vi "Single Sweep.vi"() -> ()   [LabVIEW 2016]
uses:
  Keithley 2600 Series/Public/Channel.ctl
  Keithley 2600 Series/Keithley 2600 Series.lvlib
panel:
  out "error out":errorcluster
  out "Data Array Out":dbl[](array[numeric])
  in  "End (V)":dbl
  in  "Start (V)":dbl
  in  "Current Limit (A)":dbl=0.1
  in  "Step Numbers":u32=1
  in  "VISA resource name":refnum<visa-resource-name>
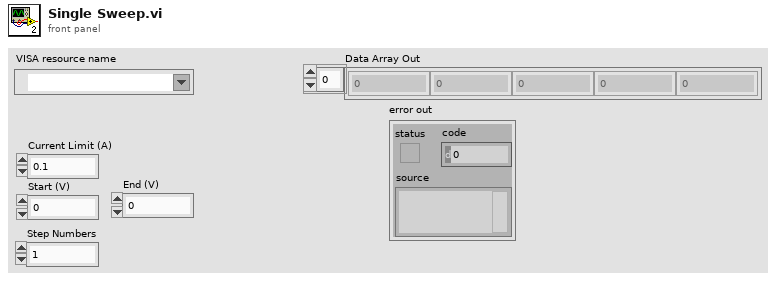
[diagram p1: front panel]
types:
  T1 = enum32{"Normal", "Big Endian", "Little Endian", "Network", "Swapped"}
  T2 = enum32{"ASCII", "Real 32", "Real 64", "Single Precision Real", "Double Precision Real"}
  T3 = enum16{"Current", "Voltage", "IV", "Resistance", "Power"}
  T4 = enum16{"Linear Current", "Linear Voltage", "Logarithimic Current", "Logarithimic Voltage", "List Current", "List Voltage"}
  T5 = typedef "Keithley 2600 Series.lvlib/Channel.ctl" = enum32{"Channel A", "Channel B"}
  T6 = enum32{"Current", "Voltage", "Resistance", "Power"}
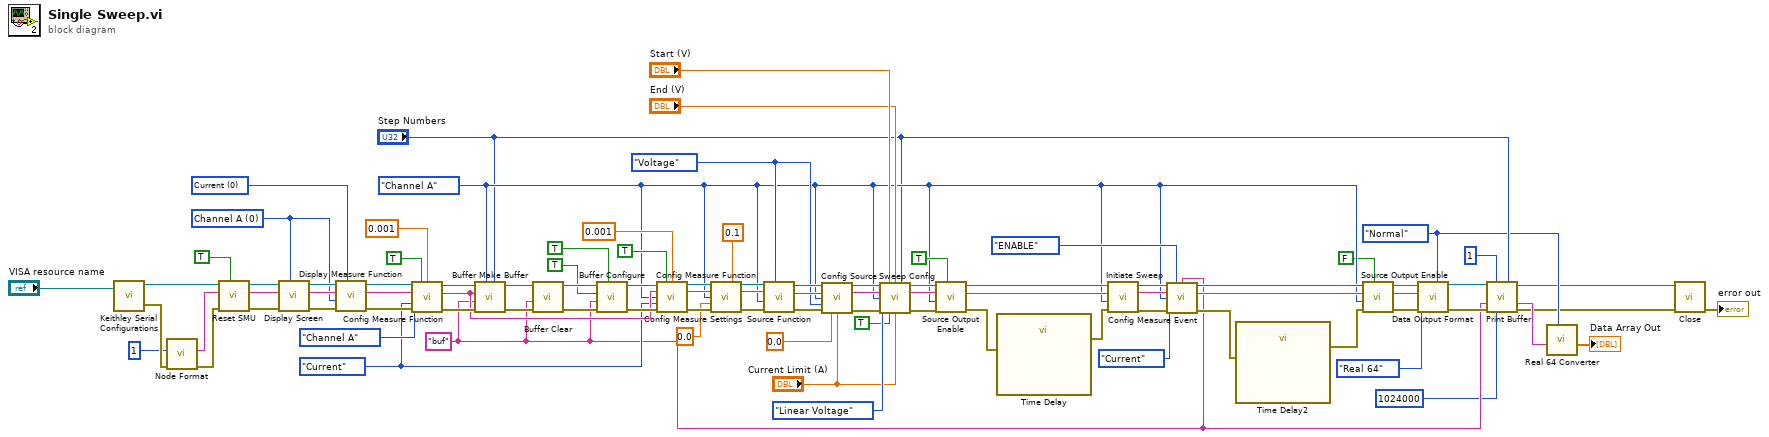
[diagram p0: block diagram]
diagram:
  w5 = T1."Normal" ("Byte Order (Normal)")
  w45 = enum32{"Current", "Voltage"}."Voltage" ("Function (Current)")
  w10 = "buf" ("Buffer Name (buf)")
  w18 = Channel."Channel A" ("Channel (Channel A)")
  w59 = T6."Current" ("Function (Current)")
  w82 = u16 0 items=["Current", "Voltage", "Resistance", "Power"] ("Function (Current)")
  w77 = u16 0 items=["Channel A", "Channel B", "Channels A & B", "User"] ("Screen (Channels A & B)")
  n1 = call "Keithley Serial Configurations.vi"("VISA resource name"="VISA resource name") -> ("error out"=w81:errorcluster, "VISA resource name out"=w90:refnum<visa-resource-name>)  [unwired: 1 in]
  n2 = call "Node Format.vi"("error in"=w81, "Node (0-64)"=i8 1) -> ("error out"=w78:errorcluster, "Formatted Node"=w79:string)  [unwired: 8 in]
  n3 = call "Reset SMU.vi"("SMU A (No)"=TRUE, "error in (no error)"=w78, "Node In"=w79, "VISA resource name"=w90) -> ("error out"=w88:errorcluster, "Node Out"=w87:string, "VISA resource name out"=w86:refnum<visa-resource-name>)  [unwired: 4 in, 1 out]
  n4 = call "Display Screen.vi"("Screen (Channels A & B)"=w77, "error in (no error)"=w88, "Node In"=w87, "VISA resource name"=w86) -> ("error out"=w85:errorcluster, "Node Out"=w84:string, "VISA resource name out"=w83:refnum<visa-resource-name>)  [unwired: 4 in, 1 out]
  n5 = call "Display Measure Function.vi"("Function (Current)"=w82, "error in (no error)"=w85, "Channel (Channel A)"=w77, "Node In"=w84, "VISA resource name"=w83) -> ("error out"=w74:errorcluster, "Node Out"=w75:string, "VISA resource name out"=w76:refnum<visa-resource-name>)  [unwired: 3 in, 1 out]
  n6 = call "Config Measure Function.vi"("VISA resource name"=w76, "Autorange (On)"=TRUE, "Low Range (1.000)"=0.001, "Node In"=w75, "Channel (Channel A)"=Channel."Channel A", "Function (Current)"=w59, "error in"=w74) -> ("VISA resource name out"=w70:refnum<visa-resource-name>, "Node Out"=w60:string, "error out"=w69:errorcluster)  [unwired: 5 in, 1 out]
  n7 = call "Buffer Make Buffer.vi"("Capacity (1)"="Step Numbers", "Channel (Channel A)"=w18, "error in (no error)"=w69, "Buffer Name (buf)"=w10, "Node In"=w60, "VISA resource name"=w70) -> ("error out"=w68:errorcluster, "VISA resource name out"=w67:refnum<visa-resource-name>)  [unwired: 2 in, 2 out]
  n8 = call "Buffer Clear.vi"("error in (no error)"=w68, "Buffer Name"=w10, "VISA resource name"=w67) -> ("error out"=w65:errorcluster, "VISA resource name out"=w66:refnum<visa-resource-name>)  [unwired: 6 in, 1 out]
  n9 = call "Buffer Configure.vi"("Collect Source Values (Off)"=TRUE, "error in (no error)"=w65, "Buffer Name"=w10, "Append Mode (Off)"=TRUE, "VISA resource name"=w66) -> ("error out"=w61:errorcluster, "VISA resource name out"=w62:refnum<visa-resource-name>)  [unwired: 4 in, 1 out]
  n10 = call "Config Measure Function.vi"("VISA resource name"=w62, "Autorange (On)"=TRUE, "Low Range (1.000)"=0.001, "Node In"=w60, "Channel (Channel A)"=w18, "Function (Current)"=w59, "error in"=w61) -> ("VISA resource name out"=w56:refnum<visa-resource-name>, "Node Out"=w55:string, "error out"=w54:errorcluster)  [unwired: 5 in, 1 out]
  n11 = call "Config Measure Settings.vi"("VISA resource name"=w56, "NPLC (1.000)"=0.1, "Node In"=w55, "Channel (Channel A)"=w18, "Measure Delay (0)"=0.0, "error in"=w54) -> ("VISA resource name out"=w49:refnum<visa-resource-name>, "Node Out"=w50:string, "error out"=w51:errorcluster)  [unwired: 6 in, 1 out]
  n12 = call "Source Function.vi"("Function (Current)"=w45, "error in (no error)"=w51, "Channel (Channel A)"=w18, "Node In"=w50, "VISA resource name"=w49) -> ("error out"=w46:errorcluster, "Node Out"=w47:string, "VISA resource name out"=w48:refnum<visa-resource-name>)  [unwired: 3 in, 1 out]
  n13 = call "Config Source.vi"("VISA resource name"=w48, "Node In"=w47, "Channel (Channel A)"=w18, "Function (Current)"=w45, "error in"=w46, "Level (0.000)"=0.0, "Limit (0.1)"="Current Limit (A)") -> ("VISA resource name out"=w43:refnum<visa-resource-name>, "Node Out"=w42:string, "error out"=w41:errorcluster)  [unwired: 5 in, 1 out]
  n14 = call "Sweep Config.vi"("VISA resource name"=w43, "Start Value"="Start (V)", "End Value"="End (V)", "Points (1)"="Step Numbers", "Node In"=w42, "Channel (Channel A)"=w18, "Sweep Type"=T4."Linear Voltage", "error in"=w41, "Sweep Mode (F: Disable)"=TRUE, "Limit (0.1)"="Current Limit (A)") -> ("VISA resource name out"=w33:refnum<visa-resource-name>, "Node Out"=w34:string, "error out"=w35:errorcluster)  [unwired: 2 in, 1 out]
  n15 = call "Source Output Enable.vi"("Output (Off)"=TRUE, "error in (no error)"=w35, "Channel (Channel A)"=w18, "Node In"=w34, "VISA resource name"=w33) -> ("error out"=w31:errorcluster, "Node Out"=w28:string, "VISA resource name out"=w30:refnum<visa-resource-name>)  [unwired: 3 in, 1 out]
  n16 = call "Time Delay"("error in (no error)"=w31) -> ("error out"=w29:errorcluster)  [unwired: 10 in]
  n17 = call "Initiate Sweep.vi"("error in"=w29, "Channel (Channel A)"=w18, "Node In"=w28, "VISA resource name"=w30) -> ("error out"=w26:errorcluster, "Node Out"=w25:string, "VISA resource name out"=w27:refnum<visa-resource-name>)  [unwired: 4 in, 1 out]
  n18 = call "Config Measure Event.vi"("VISA resource name"=w27, "Configure Measurement (Disable)"=enum8{"DISABLE", "ENABLE", "ASYNC"}."ENABLE", "Buffer 1"=w10, "Node In"=w25, "Channel (Channel A)"=w18, "Function (Current)"=T3."Current", "error in"=w26) -> ("VISA resource name out"=w21:refnum<visa-resource-name>, "Node Out"=w19:string, "error out"=w22:errorcluster)  [unwired: 5 in, 1 out]
  n19 = call "Time Delay2"("error in (no error)"=w22) -> ("error out"=w20:errorcluster)  [unwired: 10 in]
  n20 = call "Source Output Enable.vi"("Output (Off)"=FALSE, "error in (no error)"=w20, "Channel (Channel A)"=w18, "Node In"=w19, "VISA resource name"=w21) -> ("error out"=w16:errorcluster, "Node Out"=w15:string, "VISA resource name out"=w14:refnum<visa-resource-name>)  [unwired: 3 in, 1 out]
  n21 = call "Data Output Format.vi"("Byte Order (Normal)"=w5, "error in (no error)"=w16, "Data Format (ASCII)"=T2."Real 64", "Node In"=w15, "VISA resource name"=w14) -> ("error out"=w11:errorcluster, "VISA resource name out"=w12:refnum<visa-resource-name>)  [unwired: 3 in, 2 out]
  n22 = call "Print Buffer.vi"("VISA resource name"=w12, "Start Index (1)"=u32 1, "End Index (1)"="Step Numbers", "Buffer Name(s)"=w10, "error in (no error)"=w11, "Byte Count (1024)"=u32 1024000) -> ("VISA resource name out"=w3:refnum<visa-resource-name>, "Buffer Data"=w6:string, "error out"=w2:errorcluster)  [unwired: 5 in, 2 out]
  n23 = call "Real 64 Converter.vi"("Byte Order (Normal)"=w5, "Data In"=w6) -> ("Data Array Out"=→"Data Array Out":dbl[])  [unwired: 9 in]
  n24 = call "Close.vi"("error in (no error)"=w2, "VISA resource name"=w3) -> ("error out"=→"error out":errorcluster)  [unwired: 9 in]
